vi "Enums.vi"() -> ()   [LabVIEW 2024]
panel:
  in  "Path":path
  out "Numeric 2":dbl
  in  "Numeric":dbl
  in  "Month":T1(ring)
  # "Overview:\nEnum is a combination of Numeric and strings\nActs like a drop down menu.\n\nInstructions:\n 1. Select the month from the month enum.\n2. Run the VI.\n3. A pop up will be dispalyed."
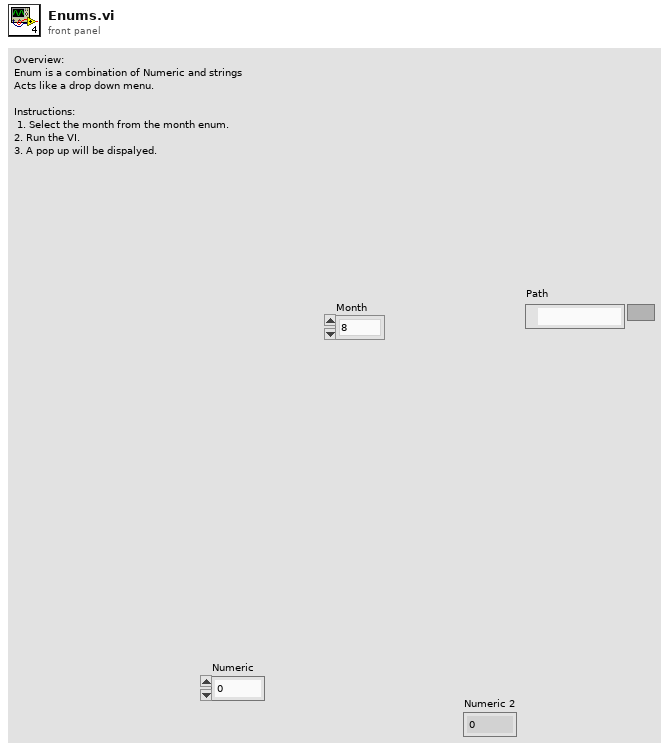
[diagram p1: front panel]
types:
  T1 = enum16{"8", "Jan", "Feb", "Mar", "Apr", "May", "Jun", "Jul", "Aug", "Sep", "Oct", "Nov", "Dec"}
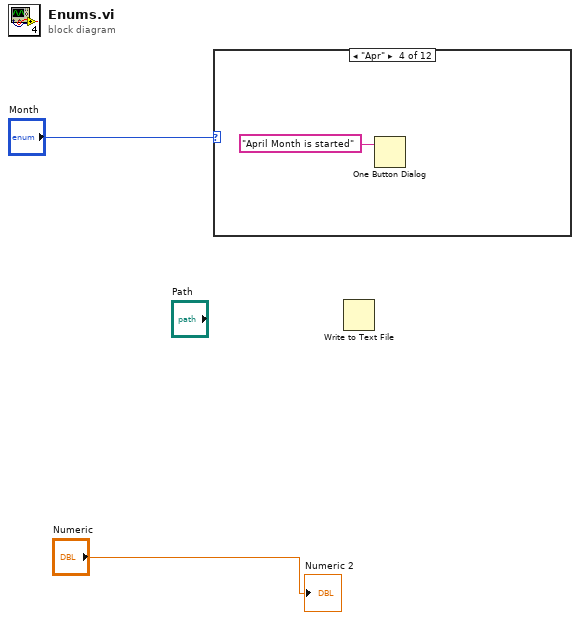
[diagram p0: block diagram]
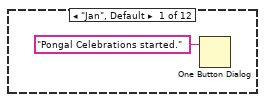
[diagram p2: hidden frame]
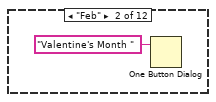
[diagram p3: hidden frame]
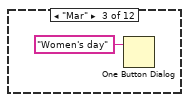
[diagram p4: hidden frame]
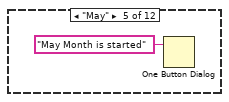
[diagram p5: hidden frame]
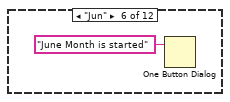
[diagram p6: hidden frame]
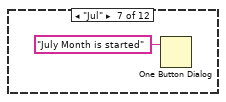
[diagram p7: hidden frame]
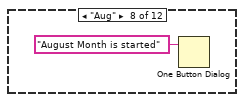
[diagram p8: hidden frame]
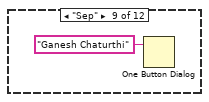
[diagram p9: hidden frame]
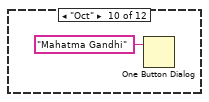
[diagram p10: hidden frame]
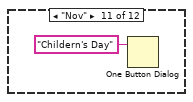
[diagram p11: hidden frame]
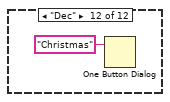
[diagram p12: hidden frame]
diagram:
  n1 = case shown="\"Apr\"" "Month" {
    frame "Jan", Default {
      n2 = One Button Dialog(message="Pongal Celebrations started.") -> ()  [unwired: 1 in, 1 out]
    }
    frame "Feb" {
      n3 = One Button Dialog(message="Valentine's Month ") -> ()  [unwired: 1 in, 1 out]
    }
    frame "Mar" {
      n4 = One Button Dialog(message="Women's day") -> ()  [unwired: 1 in, 1 out]
    }
    frame "Apr" {
      n5 = One Button Dialog(message="April Month is started") -> ()  [unwired: 1 in, 1 out]
    }
    frame "May" {
      n6 = One Button Dialog(message="May Month is started") -> ()  [unwired: 1 in, 1 out]
    }
    frame "Jun" {
      n7 = One Button Dialog(message="June Month is started") -> ()  [unwired: 1 in, 1 out]
    }
    frame "Jul" {
      n8 = One Button Dialog(message="July Month is started") -> ()  [unwired: 1 in, 1 out]
    }
    frame "Aug" {
      n9 = One Button Dialog(message="August Month is started") -> ()  [unwired: 1 in, 1 out]
    }
    frame "Sep" {
      n10 = One Button Dialog(message="Ganesh Chaturthi") -> ()  [unwired: 1 in, 1 out]
    }
    frame "Oct" {
      n11 = One Button Dialog(message="Mahatma Gandhi") -> ()  [unwired: 1 in, 1 out]
    }
    frame "Nov" {
      n12 = One Button Dialog(message="Childern's Day") -> ()  [unwired: 1 in, 1 out]
    }
    frame "Dec" {
      n13 = One Button Dialog(message="Christmas") -> ()  [unwired: 1 in, 1 out]
    }
  }
  n14 = Write to Text File() -> ()  [unwired: 4 in, 3 out]
  "Numeric 2" <- "Numeric"
